vi "read_db_for_dcs_spot.vi"(8 "error in (no error)":errorcluster, 11 "Constraints":T2) -> (0 "error out":errorcluster, 3 "Array":T1[](array[typedef]))   [LabVIEW 2012]
uses:
  DCSConstraints.ctl
  dcs_spot.ctl
  <vilib>/addons/database/Auxilliary.llb/DB Tools Cursor Type.ctl
  <vilib>/addons/database/Connection.llb/Conn Execute.vi
  <vilib>/addons/database/Recordset.llb/Rec Fetch Recordset Data (R).vi
  <vilib>/addons/database/Recordset.llb/Rec Destroy - Connection.vi
  <vilib>/addons/database/_DB Variant To Data/Database Variant To Data.xnode
  <vilib>/addons/database/NI_Database_API.lvlib
panel:
  out "resulting string":string
  out "SQL Query Sintax":string
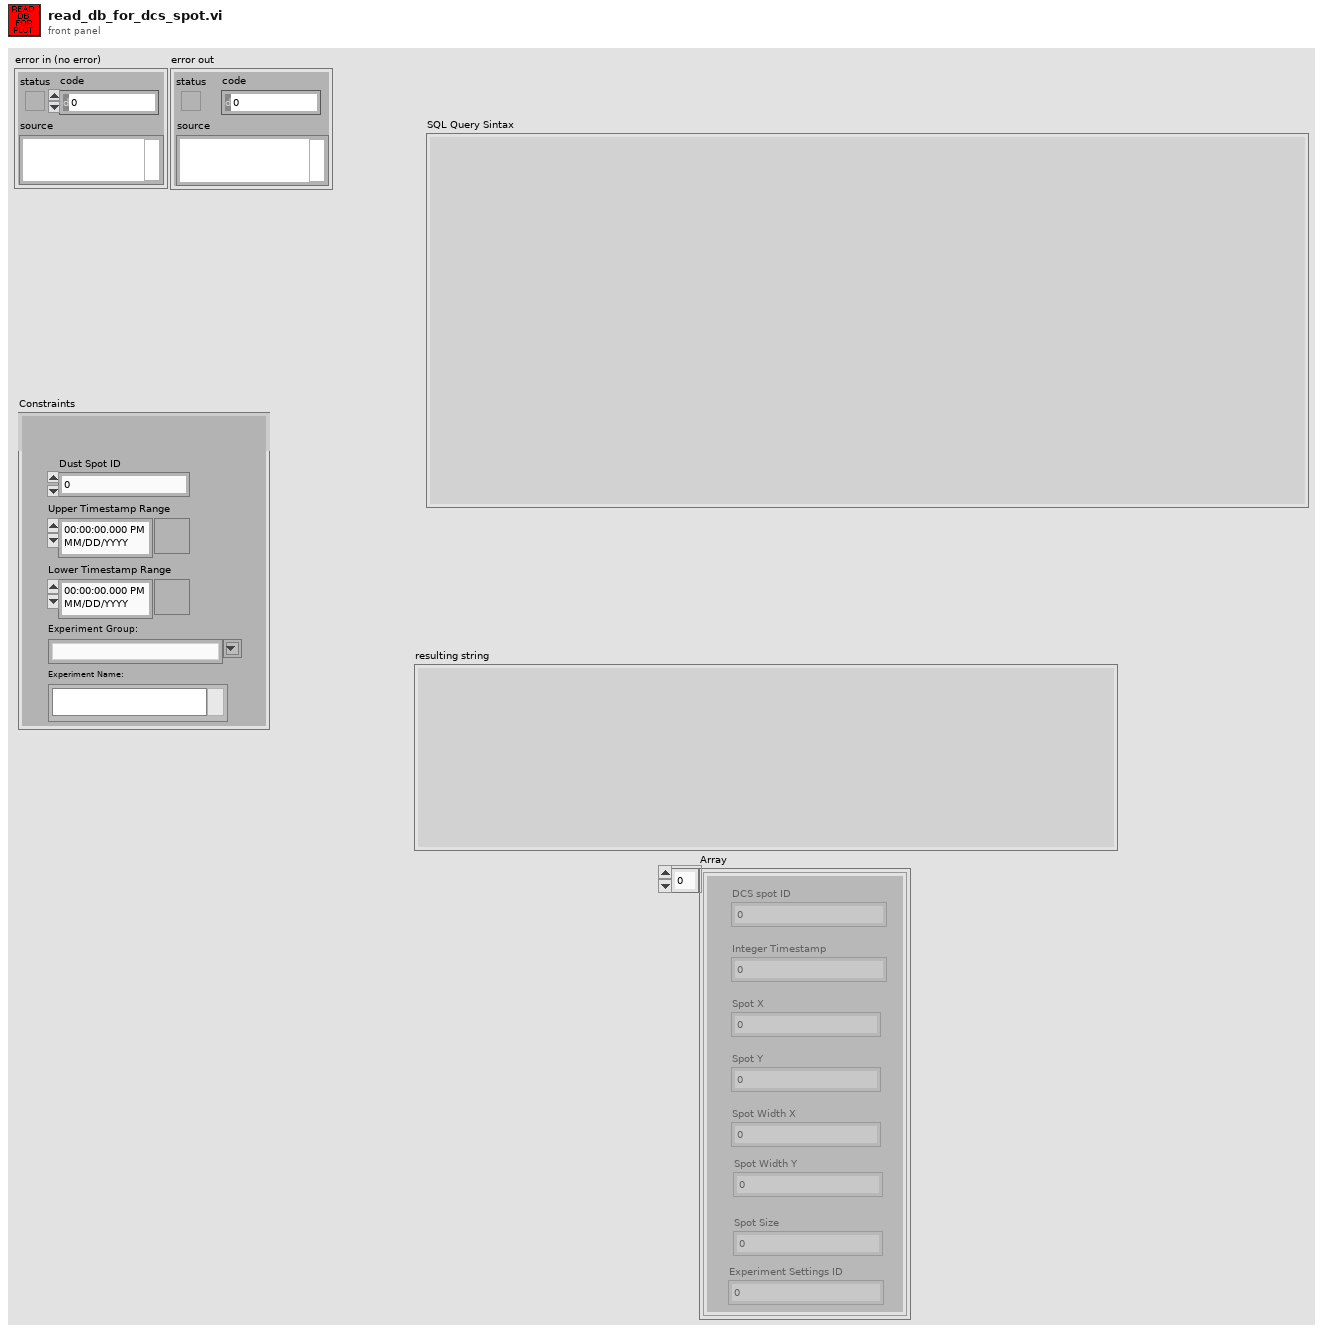
[diagram p1: front panel]
types:
  T1 = typedef "dcs_spot.ctl" = cluster{"DCS spot ID":i32, "Integer Timestamp":i64, "Spot X":dbl, "Spot Y":dbl, "Spot Width X":dbl, "Spot Width Y":dbl, "Spot Size":i32, "Experiment Settings ID":i32}
  T2 = typedef "DCSConstraints.ctl" = cluster{"Upper Timestamp Range":timestamp, "Lower Timestamp Range":timestamp, "Experiment Group:":string, "Experiment Name:":i32[], "name array":string[], "Dust Spot ID":dbl}
  T3 = typedef "NI_Database_API.lvlib/DB Tools Cursor Type.ctl" = enum16{"forward-only", "keyset", "dynamic", "static"}
  T4 = typedef "NI_Database_API.lvlib/Conn ObjectReference.ctl" = refnum<k1>
  T5 = typedef "NI_Database_API.lvlib/Rec ObjectReference.ctl" = refnum<k1>
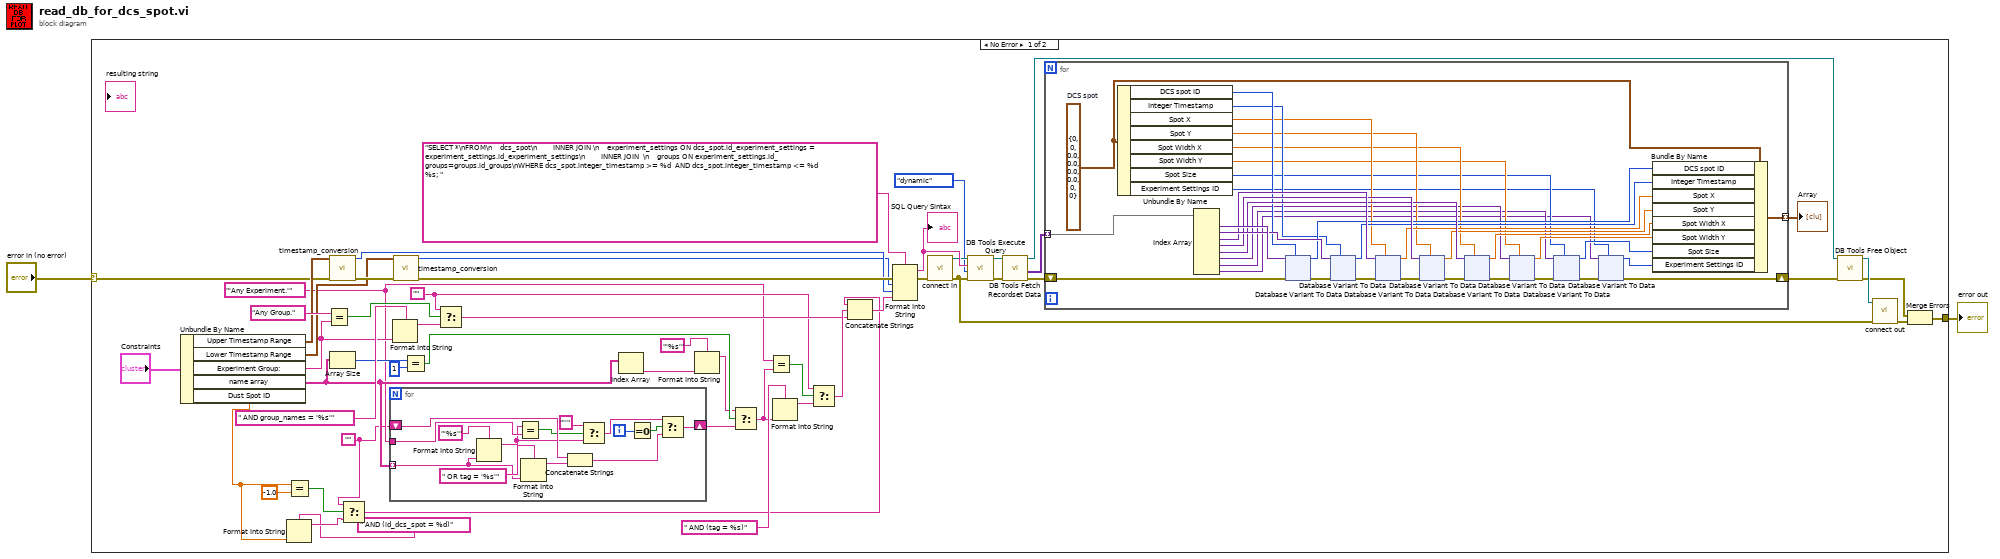
[diagram p0: block diagram]
diagram:
  n1 = case shown="No Error" "error in (no error)" {
    selector: "error in (no error)" -> [w32 w363]
    tunnel: [w16 w363] -> w1
    frame No Error {
      w8 = ""
      w37 = ""
      w20 = "'Any Experiment.'"
      n2 = Unbundle By Name("Constraints") -> ("Upper Timestamp Range"=w44:timestamp, "Lower Timestamp Range"=w45:timestamp, "Experiment Group:"=w41:string, "name array"=w25:string[], "Dust Spot ID"=w3:dbl)
      n3 = Format Into String(format string=" AND (id_dcs_spot = %d)" ("string"), w3) -> (resulting string=w7:string)  [unwired: 2 in, 1 out]
      n4 = Equal?(x=w3, y=-1.0) -> (x = y?=w9:bool)
      n5 = Equal?(x="Any Group.", y=w41) -> (x = y?=w50:bool)
      n6 = call "timestamp_conversion.vi"("error in (no error)"=w32, "Time Stamp"=w44) -> ("error out"=w49:errorcluster, "Integer Time"=w14:i64)  [unwired: 7 in]
      n7 = Array Size(array=w25) -> (size(s)=w29:i32)
      n8 = Select(t=w8, s=w9, f=w7) -> (s? t:f=w5:string)
      n9 = for {
        tunnel: w25 -> [w63] mode=indexing
        shift-right: [w65] -> w26
        shift-left: w8 -> [w70]
        tunnel: w20 -> [w61]
        i -> [w67]
        n10 = Format Into String(format string="'%s'", w63) -> (resulting string=w59:string)  [unwired: 2 in, 1 out]
        n11 = Equal?(x=w59, y=w61) -> (x = y?=w60:bool)
        n12 = Format Into String(format string=" OR tag = '%s'" ("string"), w63) -> (resulting string=w69:string)  [unwired: 2 in, 1 out]
        n13 = Concatenate Strings(w70, w69) -> (w64:string)
        n14 = Select(t="''", s=w60, f=w59) -> (s? t:f=w58:string)
        n15 = Equal To 0?(x=w67) -> (x = 0?=w66:bool)
        n16 = Select(t=w58, s=w66, f=w64) -> (s? t:f=w65:string)
      }
      n17 = Format Into String(format string=" AND group_names = '%s'" ("string"), w41) -> (resulting string=w40:string)  [unwired: 2 in, 1 out]
      n18 = call "timestamp_conversion.vi"("error in (no error)"=w49, "Time Stamp"=w45) -> ("error out"=w31:errorcluster, "Integer Time"=w12:i64)  [unwired: 7 in]
      n19 = Equal?(x=w29, y=1) -> (x = y?=w27:bool)
      n20 = Select(t=w37, s=w50, f=w40) -> (s? t:f=w46:string)
      n21 = Index Array(array=w25) -> (element=w23:string)  [unwired: 1 in]
      n22 = Format Into String(format string="'%s'", w23) -> (resulting string=w22:string)  [unwired: 2 in, 1 out]
      n23 = Select(t=w22, s=w27, f=w26) -> (s? t:f=w21:string)
      n24 = Equal?(x=w20, y=w21) -> (x = y?=w51:bool)
      n25 = Format Into String(format string=" AND (tag = %s)" ("string"), w21) -> (resulting string=w38:string)  [unwired: 2 in, 1 out]
      n26 = Select(t=w37, s=w51, f=w38) -> (s? t:f=w47:string)
      n27 = Concatenate Strings(w5, w47, w46) -> (w15:string)
      n28 = Format Into String(format string="SELECT *\nFROM\n    dcs_spot\n        INNER JOIN \n    experiment_settings ON dcs_spot.id_experiment_settings = experiment_settings.id_experiment_settings\n        INNER JOIN  \n    groups ON experiment_settings.id_groups=groups.id_groups\nWHERE dcs_spot.integer_timestamp >= %d  AND dcs_spot.integer_timestamp <= %d %s; " ("string"), error in=w31, w12, w14, w15) -> (resulting string=w34:string, error out=w30:errorcluster)  [unwired: 1 in]
      "SQL Query Sintax" <- w34
      n29 = call "connect in.vi"("error in (no error)"=w30) -> ("error out"=w11:errorcluster, "Database Connection"=w19:T4)  [unwired: 6 in, 1 out]
      n30 = call-poly <vilib>:"DB Tools Execute Query.vi"("error in (no error)"=w11, "cursor type"=DB_Tools_Cursor_Type."dynamic", "SQL query"=w34, "connection reference"=w19) -> ("error out"=w36:errorcluster, "recordset reference"=w35:T5)  [unwired: 4 in]
      n31 = call-poly <vilib>:"DB Tools Fetch Recordset Data.vi"("error in (no error)"=w36, "recordset reference"=w35) -> ("error out"=w55:errorcluster, "recordset data"=w52:variant[][], "recordset reference out"=w56:T5)  [unwired: 3 in]
      n32 = for {
        tunnel: w52 -> [w106] mode=indexing
        shift-right: [w71] -> w54
        shift-left: w55 -> [w105]
        tunnel: [w97] -> w10 mode=indexing
        w94 = T1 {"DCS spot ID"=0, "Integer Timestamp"=0, "Spot X"=0.0, "Spot Y"=0.0, "Spot Width X"=0.0, "Spot Width Y"=0.0, "Spot Size"=0, "Experiment Settings ID"=0}  # DCS spot
        n33 = Unbundle By Name(w94) -> ("DCS spot ID"=w93:i32, "Integer Timestamp"=w91:i64, "Spot X"=w89:dbl, "Spot Y"=w87:dbl, "Spot Width X"=w85:dbl, "Spot Width Y"=w81:dbl, "Spot Size"=w79:i32, "Experiment Settings ID"=w76:i32)
        n34 = Index Array(array=w106) -> (element #1=w104:variant, element #2=w103:variant, element #3=w101:variant, element #4=w99:variant, element #5=w96:variant, element #6=w82:variant, element #7=w78:variant, element #8=w75:variant)  [unwired: 8 in]
        n35 = xnode "Database Variant To Data"("database variant"=w104, "error in (no error)"=w105, "type"=w93) -> ("data"=w92:i32, "error out"=w102:errorcluster)
        n36 = xnode "Database Variant To Data"("database variant"=w103, "error in (no error)"=w102, "type"=w91) -> ("data"=w90:i64, "error out"=w100:errorcluster)
        n37 = xnode "Database Variant To Data"("database variant"=w101, "error in (no error)"=w100, "type"=w89) -> ("data"=w88:dbl, "error out"=w98:errorcluster)
        n38 = xnode "Database Variant To Data"("database variant"=w99, "error in (no error)"=w98, "type"=w87) -> ("data"=w86:dbl, "error out"=w95:errorcluster)
        n39 = xnode "Database Variant To Data"("database variant"=w96, "error in (no error)"=w95, "type"=w85) -> ("data"=w84:dbl, "error out"=w83:errorcluster)
        n40 = xnode "Database Variant To Data"("database variant"=w82, "error in (no error)"=w83, "type"=w81) -> ("data"=w80:dbl, "error out"=w73:errorcluster)
        n41 = xnode "Database Variant To Data"("database variant"=w78, "error in (no error)"=w73, "type"=w79) -> ("data"=w77:i32, "error out"=w72:errorcluster)
        n42 = xnode "Database Variant To Data"("database variant"=w75, "error in (no error)"=w72, "type"=w76) -> ("data"=w74:i32, "error out"=w71:errorcluster)
        n43 = Bundle By Name(cluster=w94, "DCS spot ID"=w92, "Integer Timestamp"=w90, "Spot X"=w88, "Spot Y"=w86, "Spot Width X"=w84, "Spot Width Y"=w80, "Spot Size"=w77, "Experiment Settings ID"=w74) -> (w97:T1)
      }
      "Array" <- w10
      n44 = call-poly <vilib>:"DB Tools Free Object.vi"("error in (no error)"=w54, "recordset reference"=w56) -> ("error out"=w18:errorcluster, "connection reference"=w53:T4)  [unwired: 8 in]
      n45 = call "connect out.vi"("error in (no error)"=w11, "connection reference"=w53) -> ("error out"=w17:errorcluster)  [unwired: 9 in]
      n46 = Merge Errors(w18, w17) -> (w16:errorcluster)
    }
    frame Error {
    }
  }
  "error out" <- w1
